vi "Controller LNLS Control FOFB Configuration Communication Loop.vi"(7 "Sync Objects":T1, 8 "error in (no error)":errorcluster, 11 "FOFB Configuration":T5={"FOFB Parameters"={"Network"={"FOFB Controller IP"="", "LNLS Control Network IP"="", "LNLS Control Network Power Supplies TCP Port"=0, "LNLS Control Network FOFB Configuration TCP Port"=0, "Data Server TCP Port"=0, "Monitoring Data TCP Port"=0, "Configuration GUI TCP Port"=0, "TCP Listening Timeout"=0}, "Fast Acquisition"={"Acquisition Period"=0, "Data Buffer Size"=0, "Monitoring Period"=0}, "Response Matrix Measurement"={"Step Amplitude"=0.0, "Time Between Steps"=0, "Step Duration"=0, "Number of Averages"=0}, "Correction Algorithm"={"Correction Period"=0, "Reference Orbit Path"=path "", "Response Matrix Path"=path "", "Correction Matrix Path"=path "", "Horizontal Correction Factor"=0.0, "Vertical Correction Factor"=0.0, "Beam Current FOFB Threshold"=0.0, "Decouple H-V"=FALSE, "Use Additional BPM LPF"=FALSE, "BPM LPF Cutoff"=0.0}, "Acquisition Network"=[], "Actuation Network"=[]}, "Number of Acquisition Chassis"=0, "Number of Actuation Chassis"=0, "Number of BPM Readings"=0, "BPM Reading Names"=[], "Selected BPM Readings"=[0, 1, 2, 3, 4, 5, 6, 7, 8, 9, 10, 11, 12, 13, 14, 15, 16, 17, 18, 19, 20, 21, 22, 23, 24, 25, 26, 27, 28, 29, 30, 31, 32, 33, 34, 35, 36, 37, 38, 39, 40, 41, 42, 43, 44, 45, 46, 47, 48, 49], "Number of Correctors"=0, "Corrector Names"=[], "Selected Correctors"=[0, 1, 2, 3, 4, 5, 6, 7, 8, 9, 10, 11, 12, 13, 14, 15, 16, 17, 18, 19, 20, 21, 22, 23, 24, 25, 26, 27, 28, 29, 30, 31, 32, 33, 34, 35, 36, 37, 38, 39, 40, 41, 42, 43, 44, 45, 46, 47, 48, 49], "Reference Orbit"=[], "Response Matrix"=[], "Correction Matrix"=[], "Acquisition Chassis Names"=[], "Actuation Chassis Names"=[], "Acquisition Variables"=[], "Actuation Variables"=[], "PS Matrix Mapping"=[], "Inverse PS Matrix Mapping"=[], "Response Matrix Beam Energy (MeV)"=0.0, "PID Parameters"=[], "BPM Planes"=[], "Corrector Planes"=[], "RMM Step Factor"=[]}) -> (0 "error out":errorcluster)   [LabVIEW 2011, in "Controller VIs.lvlib"]
uses:
  Controller VIs.lvlib
  Types Definitions/Type FOFB Configuration.ctl
  Types Definitions/Type FOFB Parameters.ctl
  Types Definitions/Type Network Configuration.ctl
  Types Definitions/Type FA Configuration.ctl
  Types Definitions/Type Response Matrix Measurement Configuration.ctl
  Types Definitions/Type Correction Algorithm Configuration.ctl
  Types Definitions/Type Acquisition Network Configuration.ctl
  Types Definitions/Type Actuation Network Configuration.ctl
  Types Definitions/Type PID Parameters.ctl
  Types Definitions/Type Synchronization Objects.ctl
  Types Definitions/Type Blocking Synchronization Objects.ctl
  Types Definitions/Type FA Request Parameters.ctl
  Types Definitions/Type BPM and PS select cluster.ctl
  Types Definitions/Type FA File Parameters.ctl
  Types Definitions/Type Monitoring Data.ctl
  Types Definitions/Type Diagnostics Data.ctl
  Types Definitions/Type CPU Loads Array.ctl
  Types Definitions/Type CPU Loads.ctl
  Types Definitions/Type Non-blocking Synchronization Objects.ctl
  Types Definitions/Type FOFB Variables.ctl
  Types Definitions/Type Actuation State.ctl
  Types Definitions/Type TCP State.ctl
  <vilib>/Platform/TimedLoop/XDataNode/timing_clust.ctl
  <vilib>/Platform/TimedLoop/XDataNode/nitl_modes.ctl
  <vilib>/Platform/TimedLoop/XDataNode/wakeup.ctl
  Controller Global Variables/LNLS Control FOFB Configuration In.vi
  <vilib>/real-time/rtutility.llb/RT Restart Target (Self).vi
  Controller Global Variables/LNLS Control FOFB Configuration Out.vi
  <vilib>/Platform/TimedLoop/XDataNode/XDataNode.xnode
  LNLS Control VIs.lvlib
  <vilib>/real-time/NI_Real-Time Libraries.lvlib
  Misc VIs.lvlib
  Controller Global Variables.lvlib
  <vilib>/Platform/TimedLoop/XDataNode/XDNodeRunTimeDep.lvlib
  Type Definitions.lvlib
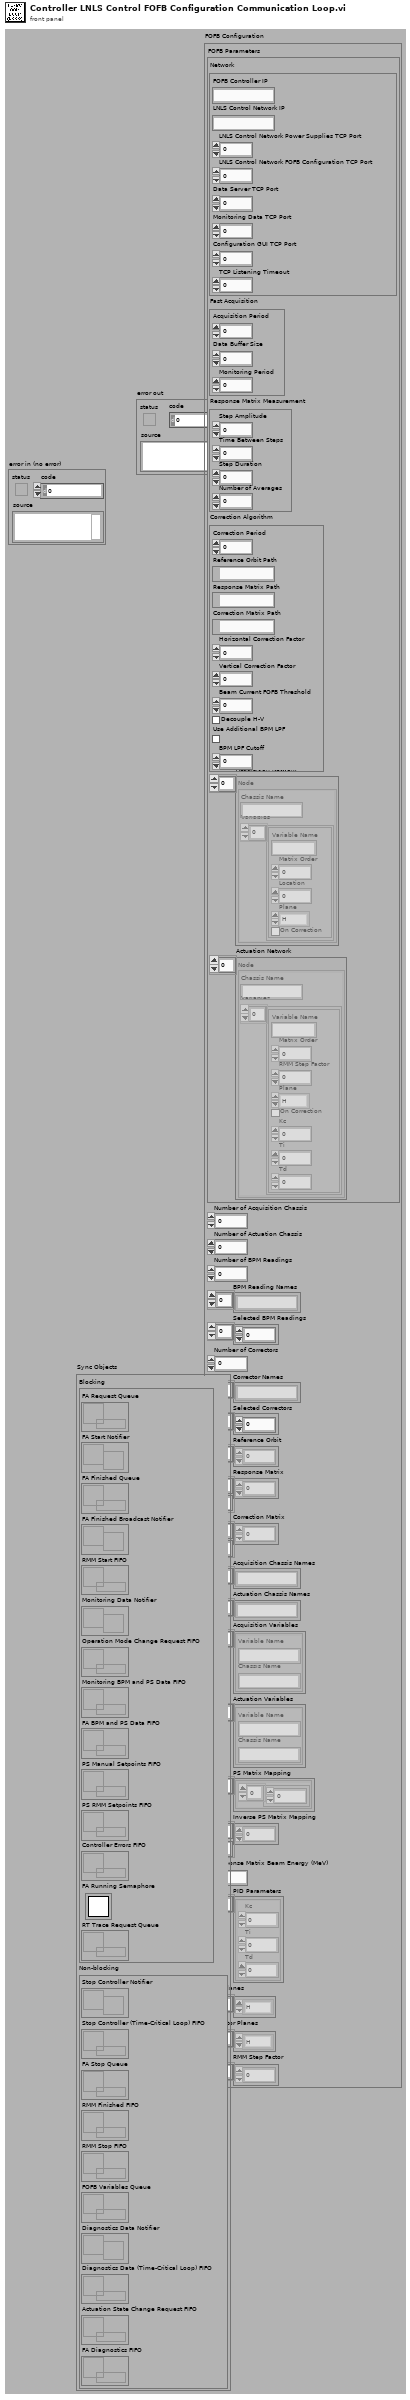
[diagram p1: front panel]
types:
  T1 = typedef "Type Definitions.lvlib/Type Synchronization Objects.ctl" = cluster{"Blocking":T2, "Non-blocking":T4}
  T2 = typedef "Type Definitions.lvlib/Type Blocking Synchronization Objects.ctl" = cluster{"FA Request Queue":refnum<queue>, "FA Start Notifier":refnum<notifier>, "FA Finished Queue":refnum<queue>, "FA Finished Broadcast Notifier":refnum<notifier>, "RMM Start FIFO":refnum<k33>, "Monitoring Data Notifier":refnum<notifier>, "Operation Mode Change Request FIFO":refnum<k33>, "Monitoring BPM and PS Data FIFO":refnum<k33>, "FA BPM and PS Data FIFO":refnum<k33>, "PS Manual Setpoints FIFO":refnum<k33>, "PS RMM Setpoints FIFO":refnum<k33>, "Controller Errors FIFO":refnum<k33>, "FA Running Semaphore":T3, "RT Trace Request Queue":refnum<queue>}
  T3 = typedef "Semaphore RefNum" = refnum<k1>
  T4 = typedef "Type Definitions.lvlib/Type Non-blocking Synchronization Objects.ctl" = cluster{"Stop Controller Notifier":refnum<notifier>, "Stop Controller (Time-Critical Loop) FIFO":refnum<k33>, "FA Stop Queue":refnum<queue>, "RMM Finished FIFO":refnum<k33>, "RMM Stop FIFO":refnum<k33>, "FOFB Variables Queue":refnum<queue>, "Diagnostics Data Notifier":refnum<notifier>, "Diagnostics Data (Time-Critical Loop) FIFO":refnum<k33>, "Actuation State Change Request FIFO":refnum<k33>, "FA Diagnostics FIFO":refnum<k33>}
  T5 = typedef "Type Definitions.lvlib/Type FOFB Configuration.ctl" = cluster{"FOFB Parameters":T6, "Number of Acquisition Chassis":i32, "Number of Actuation Chassis":i32, "Number of BPM Readings":i32, "BPM Reading Names":string[], "Selected BPM Readings":u32[], "Number of Correctors":i32, "Corrector Names":string[], "Selected Correctors":u32[], "Reference Orbit":dbl[], "Response Matrix":dbl[][], "Correction Matrix":dbl[][], "Acquisition Chassis Names":string[], "Actuation Chassis Names":string[], "Acquisition Variables":cluster{"Variable Name":string, "Chassis Name":string}[], "Actuation Variables":cluster{"Variable Name":string, "Chassis Name":string}[], "PS Matrix Mapping":cluster{u32[]}[], "Inverse PS Matrix Mapping":u32[][], "Response Matrix Beam Energy (MeV)":dbl, "PID Parameters":T13[], "BPM Planes":enum8{"H", "V"}[], "Corrector Planes":enum8{"H", "V"}[], "RMM Step Factor":dbl[]}
  T6 = typedef "Type Definitions.lvlib/Type FOFB Parameters.ctl" = cluster{"Network":T7, "Fast Acquisition":T8, "Response Matrix Measurement":T9, "Correction Algorithm":T10, "Acquisition Network":T11, "Actuation Network":T12}
  T7 = typedef "Type Definitions.lvlib/Type Network Configuration.ctl" = cluster{"FOFB Controller IP":string, "LNLS Control Network IP":string, "LNLS Control Network Power Supplies TCP Port":u16, "LNLS Control Network FOFB Configuration TCP Port":u16, "Data Server TCP Port":u16, "Monitoring Data TCP Port":u16, "Configuration GUI TCP Port":u16, "TCP Listening Timeout":i32}
  T8 = typedef "Type Definitions.lvlib/Type FA Configuration.ctl" = cluster{"Acquisition Period":u32, "Data Buffer Size":u32, "Monitoring Period":u32}
  T9 = typedef "Type Definitions.lvlib/Type Response Matrix Measurement Configuration.ctl" = cluster{"Step Amplitude":dbl, "Time Between Steps":u32, "Step Duration":u32, "Number of Averages":u32}
  T10 = typedef "Type Definitions.lvlib/Type Correction Algorithm Configuration.ctl" = cluster{"Correction Period":u32, "Reference Orbit Path":path, "Response Matrix Path":path, "Correction Matrix Path":path, "Horizontal Correction Factor":dbl, "Vertical Correction Factor":dbl, "Beam Current FOFB Threshold":dbl, "Decouple H-V":bool, "Use Additional BPM LPF":bool, "BPM LPF Cutoff":dbl}
  T11 = typedef "Type Definitions.lvlib/Type Acquisition Network Configuration.ctl" = cluster{"Chassis Name":string, "Variables":cluster{"Variable Name":string, "Matrix Order":u32, "Location":dbl, "Plane":enum8{"H", "V"}, "On Correction":bool}[]}[]
  T12 = typedef "Type Definitions.lvlib/Type Actuation Network Configuration.ctl" = cluster{"Chassis Name":string, "Variables":cluster{"Variable Name":string, "Matrix Order":u32, "RMM Step Factor":dbl, "Plane":enum8{"H", "V"}, "On Correction":bool, "Kc":dbl, "Ti":dbl, "Td":dbl}[]}[]
  T13 = typedef "Type Definitions.lvlib/Type PID Parameters.ctl" = cluster{"Kc":fxp<+/-,16,8>, "Ti":fxp<+/-,16,8>, "Td":fxp<+/-,16,8>}
  T14 = enum16{"Idle Mode", "Error Mode", "Manual Mode", "FOFB Mode", "RMM Mode"}
  T15 = typedef "Type Definitions.lvlib/Type TCP State.ctl" = enum16{"Idle", "Wait Connection", "Read Data", "Process Data", "Write Data", "Close Connection"}
  T16 = typedef "XDNodeRunTimeDep.lvlib/timing_clust.ctl" = cluster{"Expected End [f-1]":u64, "Actual End [f-1]":u64, "Finished Late? [f-1]":bool, "Expected End [i-1]":u64, "Actual End [i-1]":u64, "Finished Late? [i-1]":bool, "Expected Start [i]":u64, "Actual Start [i]":u64, "Expected Start [f]":u64, "Actual Start [f]":u64, "Source Name":string, "Structure Name":string, "Period":i64, "Deadline":i64, "Offset":i64, "Start":i64, "Priority":i32, "Timeout":i32, "Mode":T17, "Wakeup Reason":T18, "Error":errorcluster, "Source Type":string, "Secondary Source Type":string, "Global End Time":u64, "Global Start Time":u64, "Frame Duration":u64, "Iteration Duration":u64, "Assigned CPU":i32, "I/O Scan Engine Mode":u32}
  T17 = typedef "XDNodeRunTimeDep.lvlib/nitl_modes.ctl" = enum32{"No Change", "Process missed periods, maintain original phase", "Discard missed periods, maintain original phase", "Process missed periods, ignore original phase", "Discard missed periods, ignore original phase"}
  T18 = typedef "XDNodeRunTimeDep.lvlib/wakeup.ctl" = enum32{"Normal", "Aborted", "Asynchronous wakeup", "Timing source error", "Timed loop error", "Timeout"}
  T19 = cluster{"Operation Mode":enum16{"Idle Mode", "Error Mode", "Manual Mode", "FOFB Mode", "RMM Mode"}, "Correction Period (usec)":i32, "Beam Energy (MeV)":sgl, "Beam Current (mA)":sgl}
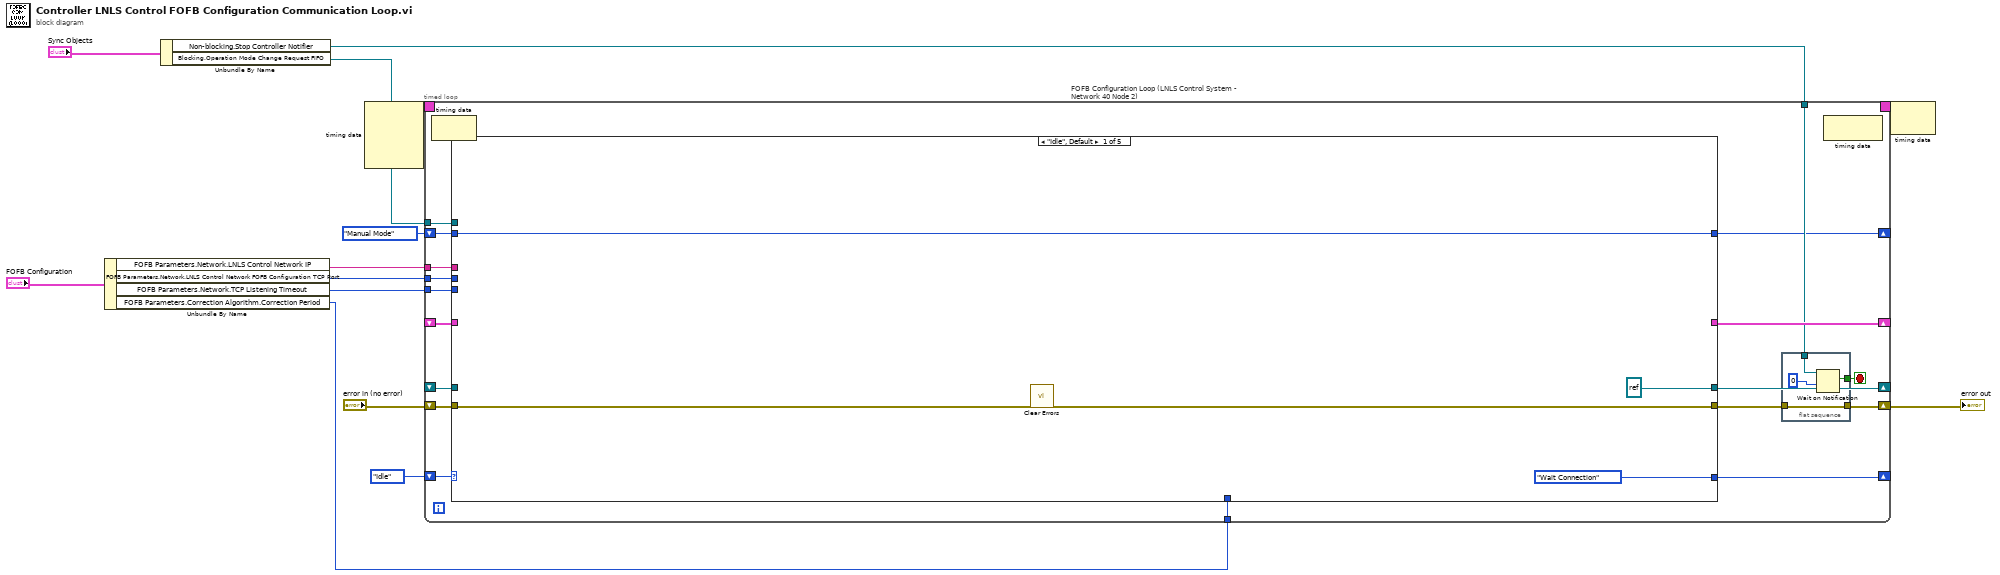
[diagram p0: block diagram]
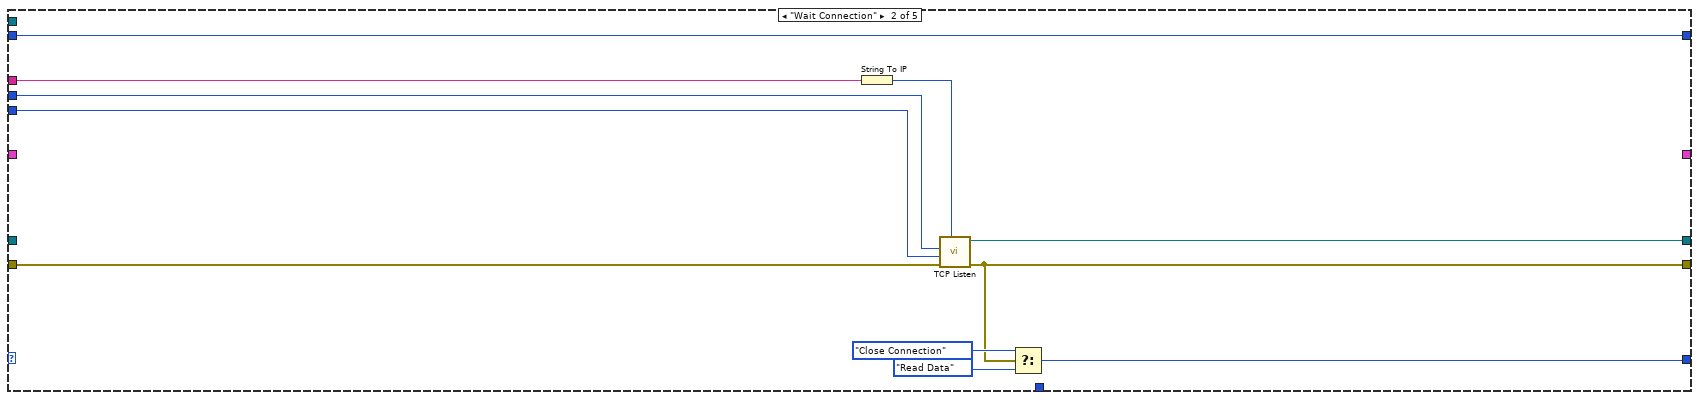
[diagram p2: hidden frame]
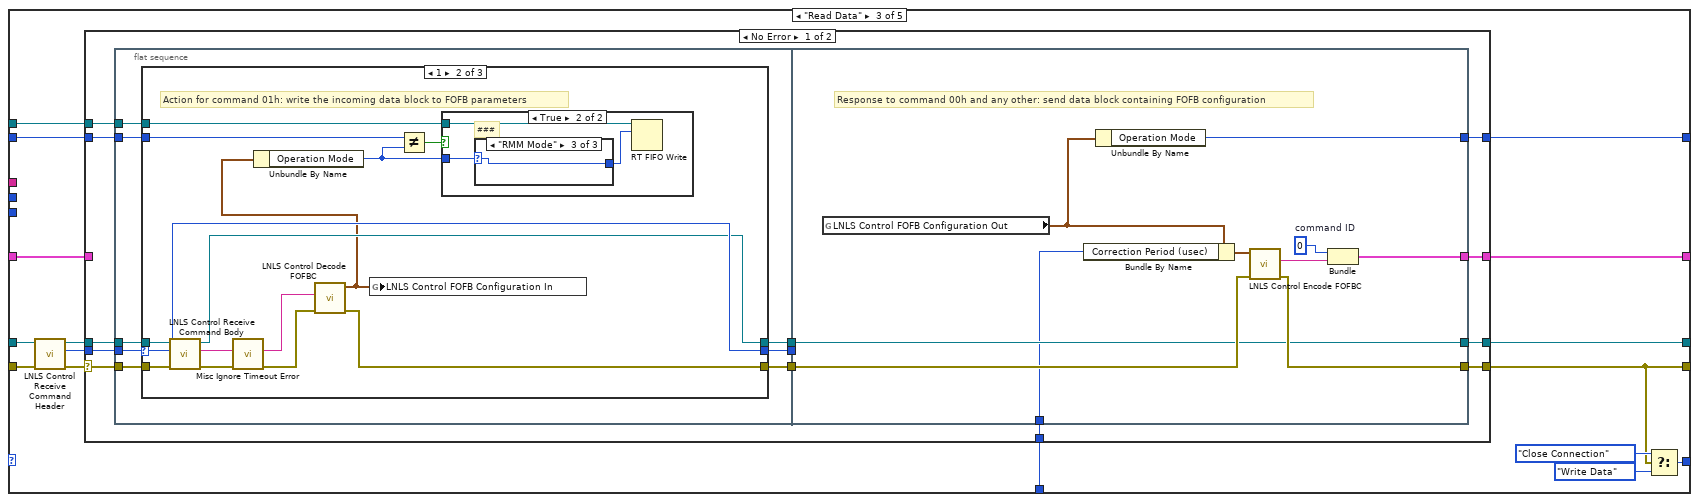
[diagram p3: hidden frame]
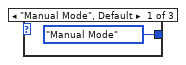
[diagram p6: hidden frame]
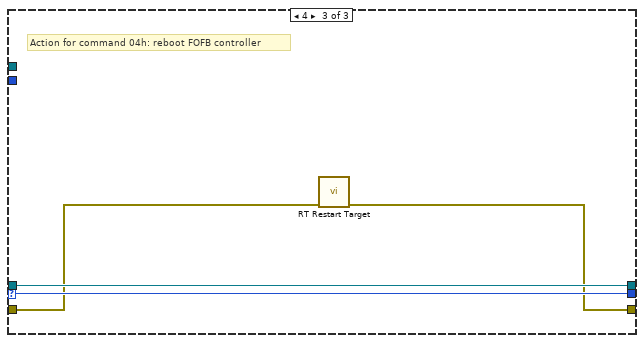
[diagram p8: hidden frame]
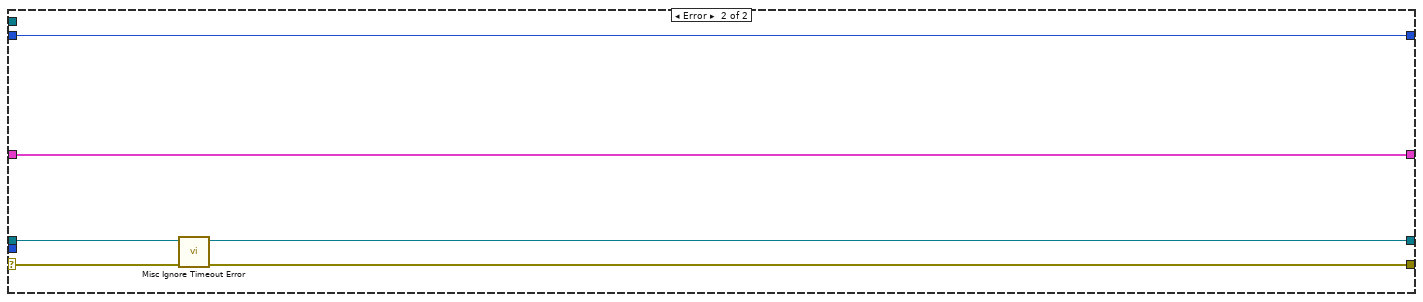
[diagram p9: hidden frame]
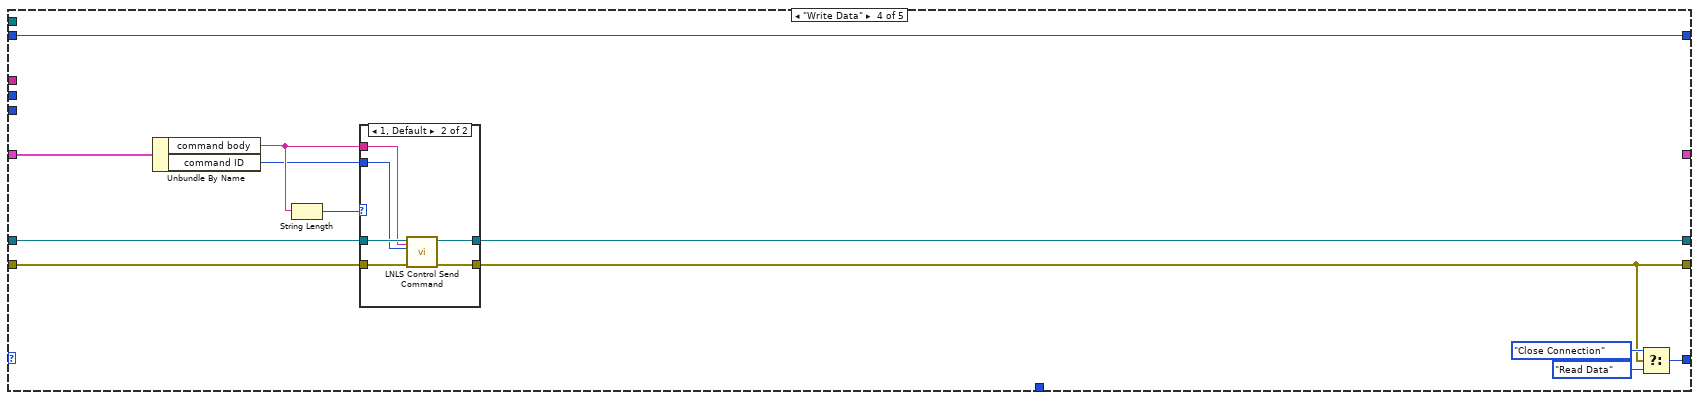
[diagram p10: hidden frame]
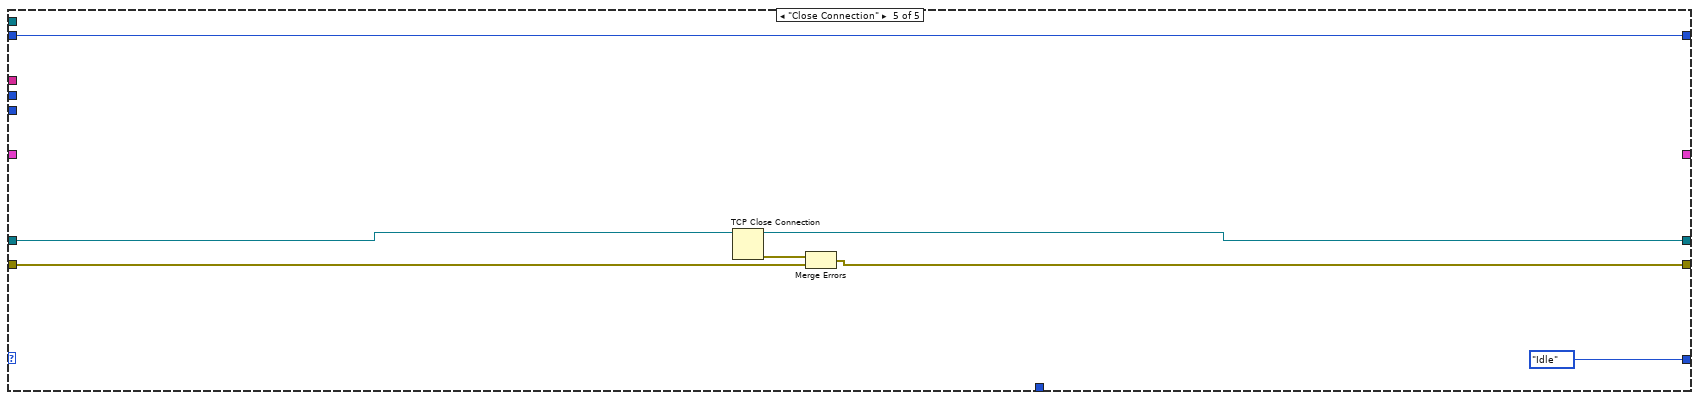
[diagram p12: hidden frame]
diagram:
  n1 = Unbundle By Name("FOFB Configuration") -> ("FOFB Parameters.Network.LNLS Control Network IP"=w9:string, "FOFB Parameters.Network.LNLS Control Network FOFB Configuration TCP Port"=w8:u16, "FOFB Parameters.Network.TCP Listening Timeout"=w6:i32, "FOFB Parameters.Correction Algorithm.Correction Period"=w1:u32)
  n2 = Unbundle By Name("Sync Objects") -> ("Non-blocking.Stop Controller Notifier"=w7:refnum<notifier>, "Blocking.Operation Mode Change Request FIFO"=w5:refnum<k33>)
  n3 = node-c288() -> (w3:T16)  [unwired: 4 in]
  n4 = timed-loop "FOFB Configuration Loop (LNLS Control System - Network 40 Node 2)" {
    shift-right: [w30] -> _
    shift-left: Type_TCP_State."Idle" ("f") -> [w32]
    shift-right: [w31] -> _
    shift-left: _ -> [w29]
    shift-right: [w19] -> w12
    shift-left: "error in (no error)" -> [w26]
    shift-right: [w28] -> _
    shift-left: _ -> [w27]
    tunnel: w9 -> [w25]
    tunnel: w8 -> [w24]
    tunnel: w7 -> [w22]
    tunnel: w6 -> [w21]
    tunnel: w5 -> [w18]
    shift-right: [w16] -> _
    shift-left: T14."Manual Mode" ("Operation Mode") -> [w17]
    timing: w3 -> [_]
    timing-out: [_] -> w2
    tunnel: w1 -> [w15]
    stop <- w23 stop-if-true
    n5 = node-c288() -> ()  [unwired: 1 in, 1 out]
    n6 = case shown="\"Idle\", Default" w32 {
      tunnel: [refnum<k5> refnum ("connection ID") w47 w66 w131 w154] -> w31
      tunnel: [w35 w40 w56 w133 w149] -> w20
      tunnel: [Type_TCP_State."Wait Connection" w50 w65 w138 Type_TCP_State."Idle"] -> w30
      tunnel: w29 -> [_ _ w63 w132 w155]
      tunnel: w26 -> [w36 w41 w64 w134 w150]
      tunnel: [_ _ w60 _ _] -> w28
      tunnel: w27 -> [_ _ w58 w130 _]
      tunnel: w25 -> [_ w45 _ _ _]
      tunnel: w24 -> [_ w44 _ _ _]
      tunnel: w21 -> [_ w43 _ _ _]
      tunnel: w18 -> [_ _ w54 _ _]
      tunnel: w17 -> [w37 w42 w53 w129 w152]
      tunnel: [w37 w42 w52 w129 w152] -> w16
      tunnel: w15 -> [_ _ w51 _ _]
      frame "Idle", Default {
        n7 = call <vilib>:"Clear Errors.vi"("error in (no error)"=w36) -> ("error out"=w35:errorcluster)  [unwired: 6 in]
      }
      frame "Wait Connection" {
        n8 = String To IP(1:w45) -> (0:w46:u32)
        n9 = call <vilib>:"TCP Listen.vi"("net address"=w46, "error in (no error)"=w41, "timeout ms (wait forever: -1)"=w43, "port"=w44) -> ("error out"=w40:errorcluster, "connection ID"=w47:refnum<k5>)  [unwired: 3 in, 3 out]
        n10 = Select(t=Type_TCP_State."Close Connection", s=w40, f=Type_TCP_State."Read Data") -> (s? t:f=w50:T15)
      }
      frame "Read Data" {
        n11 = call "LNLS Control Receive Command Header.vi"("error in (no error)"=w64, "connection ID"=w63) -> ("error out"=w59:errorcluster, "command ID"=w55:u8, "connection ID out"=w62:refnum<k5>)  [unwired: 7 in]
        n12 = case shown="No Error" w59 {
          selector: w59 -> [w74 w126]
          tunnel: [w79 w128] -> w66
          tunnel: [w78 w125] -> w56
          tunnel: w62 -> [w77 w128]
          tunnel: w55 -> [w76 _]
          tunnel: [w75 w127] -> w60
          tunnel: w58 -> [_ w127]
          tunnel: w54 -> [w70 _]
          tunnel: w53 -> [w69 w124]
          tunnel: [w68 w124] -> w52
          tunnel: w51 -> [w67 _]
          frame No Error {
            n13 = flat-sequence {
              tunnel: [w87] -> w73
              tunnel: [w86] -> w72
              tunnel: w77 -> [w85]
              tunnel: w76 -> [w84]
              tunnel: w74 -> [w83]
              tunnel: [w82] -> w71
              tunnel: w70 -> [w81]
              tunnel: w69 -> [w80]
              tunnel: [w121] -> w79
              tunnel: w73 -> [w121]
              tunnel: [w123] -> w78
              tunnel: w72 -> [w122]
              tunnel: [w120] -> w75
              tunnel: w71 -> [_]
              tunnel: [w114] -> w68
              tunnel: w67 -> [w116]
              frame #0 {
                n14 = case shown="1" w84 {
                  selector: w84 -> [w88 w99 w113]
                  tunnel: w83 -> [w90 w102 w111]
                  tunnel: [w90 w100 w110] -> w86
                  tunnel: [w89 w98 w112] -> w87
                  tunnel: w85 -> [w89 w103 w112]
                  tunnel: [w88 w99 w113] -> w82
                  tunnel: w81 -> [_ w95 _]
                  tunnel: w80 -> [_ w94 _]
                  frame 0, Default {
                  }
                  frame 1 {
                    # "Action for command 01h: write the incoming data block to FOFB parameters"
                    n15 = call "LNLS Control Receive Command Body.vi"("error in (no error)"=w102, "connection ID"=w103) -> ("error out"=w97:errorcluster, "command body"=w101:string, "connection ID out"=w98:refnum<k5>)  [unwired: 6 in, 1 out]
                    n16 = call "Misc Ignore Timeout Error.vi"("error in (no error)"=w97) -> ("error out"=w96:errorcluster)  [unwired: 10 in]
                    n17 = call "LNLS Control Decode FOFBC.vi"("error in (no error)"=w96, "command body"=w101) -> ("error out"=w100:errorcluster, "LNLS Control FOFB Configuration"=w91:T19)  [unwired: 8 in]
                    n18 = Unbundle By Name(w91) -> ("Operation Mode"=w92:T14)
                    n19 = global write "LNLS Control FOFB Configuration In.vi" "LNLS Control FOFB Configuration In"(w91) -> ()
                    n20 = Not Equal?(x=w94, y=w92) -> (x != y?=w93:bool)
                    n21 = case shown="True" w93 {
                      tunnel: w95 -> [_ w106]
                      tunnel: w92 -> [_ w105]
                      frame False {
                      }
                      frame True {
                        # "###"
                        n22 = case shown="\"RMM Mode\"" w105 {
                          selector: w105 -> [_ w108 w109]
                          tunnel: [T14."Manual Mode" ("Operation Mode") w108 w109] -> w104
                          frame "Manual Mode", Default {
                          }
                          frame "FOFB Mode" {
                          }
                          frame "RMM Mode" {
                          }
                        }
                        n23 = RT FIFO Write(0:w106, 1:w104) -> ()  [unwired: 3 in, 4 out]
                      }
                    }
                  }
                  frame 4 {
                    # "Action for command 04h: reboot FOFB controller"
                    n24 = call-poly <vilib>:"RT Restart Target.vi"("error in (no error)"=w111) -> ("error out"=w110:errorcluster)  [unwired: 10 in]
                  }
                }
              }
              frame #1 {
                w118 = u8 0  # command ID
                # "Response to command 00h and any other: send data block containing FOFB configuration"
                n25 = global read "LNLS Control FOFB Configuration Out.vi" "LNLS Control FOFB Configuration Out"() -> (w115:T19)
                n26 = Bundle By Name(cluster=w115, "Correction Period (usec)"=w116) -> (w117:T19)
                n27 = Unbundle By Name(w115) -> ("Operation Mode"=w114:T14)
                n28 = call "LNLS Control Encode FOFBC.vi"("error in (no error)"=w122, "LNLS Control FOFB Configuration"=w117) -> ("error out"=w123:errorcluster, "command body"=w119:string)  [unwired: 8 in]
                n29 = Bundle("command ID"=w118, "command body"=w119) -> (w120:cluster{"command ID":u8, "command body":string})  [unwired: 1 in]
              }
            }
          }
          frame Error {
            n30 = call "Misc Ignore Timeout Error.vi"("error in (no error)"=w126) -> ("error out"=w125:errorcluster)  [unwired: 10 in]
          }
        }
        n31 = Select(t=Type_TCP_State."Close Connection", s=w56, f=Type_TCP_State."Write Data") -> (s? t:f=w65:T15)
      }
      frame "Write Data" {
        n32 = Unbundle By Name(w130) -> ("command body"=w137:string, "command ID"=w135:u8)
        n33 = String Length(string=w137) -> (length=w136:i32)
        n34 = case shown="1, Default" w136 {
          tunnel: w132 -> [w141 w148]
          tunnel: w134 -> [w142 w147]
          tunnel: [w142 w146] -> w133
          tunnel: [w141 w145] -> w131
          tunnel: w137 -> [_ w144]
          tunnel: w135 -> [_ w143]
          frame 0 {
          }
          frame 1, Default {
            n35 = call "LNLS Control Send Command.vi"("command body"=w144, "error in (no error)"=w147, "command ID"=w143, "connection ID"=w148) -> ("error out"=w146:errorcluster, "connection ID out"=w145:refnum<k5>)  [unwired: 6 in]
          }
        }
        n36 = Select(t=Type_TCP_State."Close Connection", s=w133, f=Type_TCP_State."Read Data") -> (s? t:f=w138:T15)
      }
      frame "Close Connection" {
        n37 = TCP Close Connection(connection ID=w155) -> (connection ID out=w154:refnum<k5>, error out=w151:errorcluster)  [unwired: 2 in]
        n38 = Merge Errors(w151, w150) -> (w149:errorcluster)
      }
    }
    n39 = flat-sequence {
      tunnel: [w158] -> w23
      tunnel: w22 -> [w157]
      tunnel: w20 -> [w156]
      tunnel: [w156] -> w19
      frame #0 {
        n40 = Wait on Notification(notifier=w157, timeout in ms (-1)=0) -> (notification=w158:bool)  [unwired: 2 in, 3 out]
      }
    }
    n41 = node-c288() -> ()  [unwired: 1 in, 1 out]
  }
  "error out" <- w12
  n42 = node-c288(w2) -> ()  [unwired: 1 out]
